vi "testVoteCount.vi"(8 "error in (no error)":errorcluster, 11 "TestCase in":refnum<class "TestVoting.lvclass">) -> (0 "error out":errorcluster, 3 "TestCase out":refnum<class "TestVoting.lvclass">)   [LabVIEW 2019, in "TestVoting.lvclass"]
uses:
  TestVoting.lvclass
  <vilib>/addons/_JKI Toolkits/VI Tester/TestCase.llb/TestCase.lvclass
  C:/Program Files (x86)/National Instruments/LabVIEW 2019/vi.lib/addons/_JKI Toolkits/VI Tester/TestCase.llb/TestCase.lvclass
panel:
  out "Vote Count":cluster{string, i32}[](array[cluster])
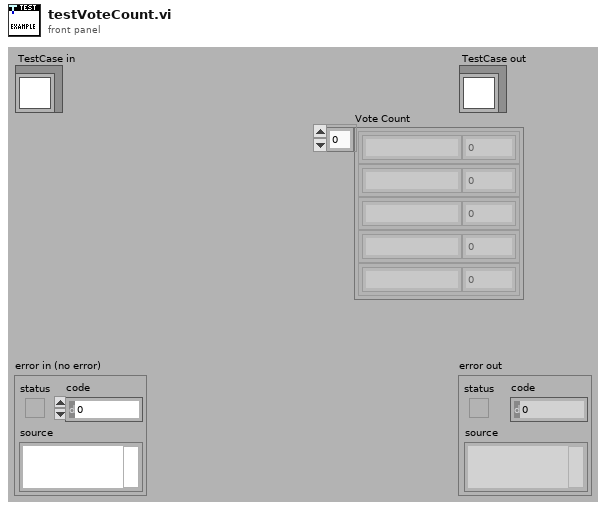
[diagram p1: front panel]
types:
  T1 = map{i32, cluster{"VoterName":string, "Ballot":string}}
  T2 = typedef "Vote Result.ctl" = cluster{"Vote":string, "Count":i32}
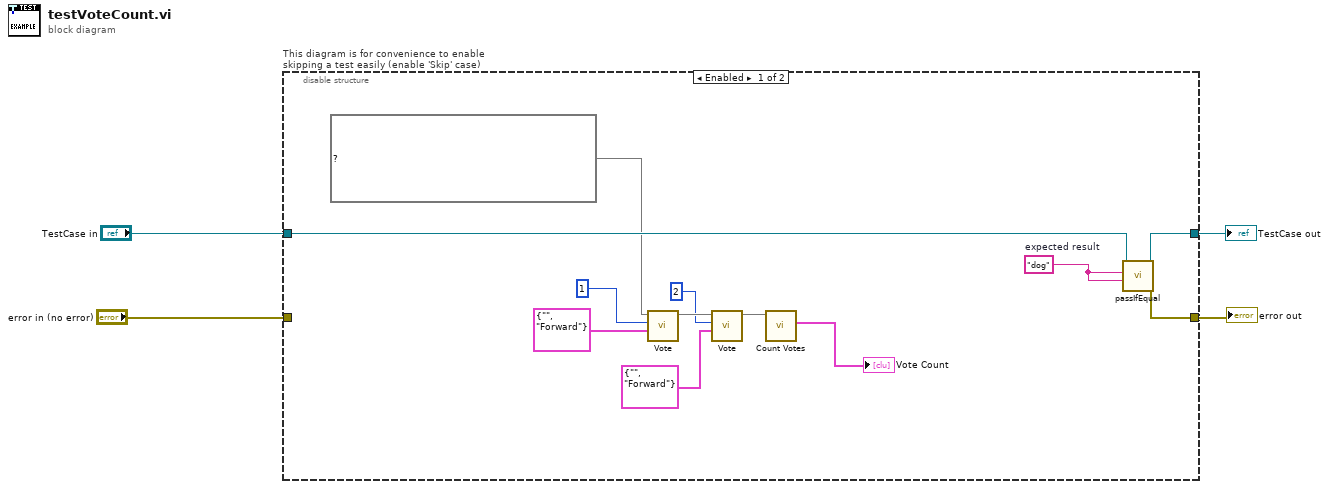
[diagram p0: block diagram]
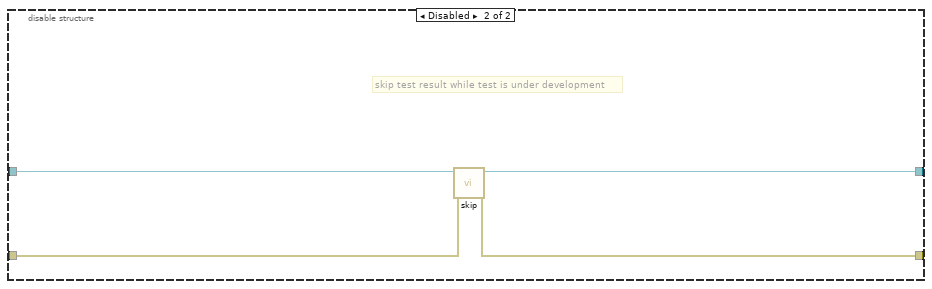
[diagram p2: hidden frame]
diagram:
  n1 = disable-structure "This diagram is for convenience to enable skipping a test easily (enable 'Skip' case)" shown="Enabled" {
    disable-tunnel: "TestCase in" -> [w16 w20]
    disable-tunnel: [w15 w18] -> w1
    disable-tunnel: [w14 w19] -> w3
    disable-tunnel: "error in (no error)" -> [_ w17]
    frame Enabled {
      w13 = "dog"  # expected result
      n2 = call "Vote.vi"("VoterInfo"=cluster{"VoterName":string, "Ballot":string} {"VoterName"="", "Ballot"="Forward"}, "VoterID"=1, "map in"=T1 {1={"VoterName"="Sam", "Ballot"=""}, 2={"VoterName"="John", "Ballot"=""}} ("map out")) -> ("map out"=w8:T1)  [unwired: 8 in]
      n3 = call "Vote.vi"("VoterInfo"=cluster{"VoterName":string, "Ballot":string} {"VoterName"="", "Ballot"="Forward"}, "VoterID"=2, "map in"=w8) -> ("map out"=w7:T1)  [unwired: 8 in]
      n4 = call "Count Votes.vi"("map in"=w7) -> ("Vote Count"=→"Vote Count":T2[])  [unwired: 9 in, 1 out]
      n5 = call-dynamic "passIfEqual.vi"("y"=w13, "x"=w13, "TestCase in"=w16) -> ("error out"=w14:errorcluster, "TestCase out"=w15:refnum<class "TestVoting.lvclass">)  [unwired: 7 in]
    }
    frame Disabled {
      # "skip test result while test is under development"
      n6 = call <vilib>:"skip.vi"("error in (no error)"=w17, "TestCase in"=w20) -> ("error out"=w19:errorcluster, "TestCase out"=w18:refnum<class "TestVoting.lvclass">)  [unwired: 8 in]
    }
  }
  "error out" <- w3
  "TestCase out" <- w1
